vi "Test Person Updates Status on Trigger Broadcast.vi"(8 "error in (no error)":errorcluster, 11 "Person Test In":refnum<class "Person Test.lvclass">) -> (0 "error out":errorcluster, 3 "Person Test Out":refnum<class "Person Test.lvclass">)   [LabVIEW 2020, in "Person Test.lvclass"]
uses:
  Person Test.lvclass
  C:/Program Files (x86)/National Instruments/LabVIEW 2020/vi.lib/Asteme/LUnit/Test Case.lvclass
  <vilib>/Asteme/Triarc Framework/Process/Process.lvclass/Process.ctl
  <vilib>/Asteme/LUnit/Test Case.lvclass/Test Case.ctl
  <vilib>/Asteme/LUnit/LUnit Assertion Result.lvclass/LUnit Assertion Result.ctl
  <vilib>/Asteme/Triarc Framework/Process/Protected/Messaging/Enqueue Message.vi
  <vilib>/Asteme/Triarc Framework/Process/Private/SubVIs/Wait for finish.vi
  <vilib>/Asteme/Triarc Framework/Process/Private/SubVIs/Set Lifecycle State.vi
  <vilib>/Asteme/Triarc Framework/Process/Public/Lifecycle/Get Lifecycle State.vi
  <vilib>/Asteme/Triarc Framework Test Suite/Support/Execution timer.vi
  <vilib>/Asteme/LUnit/Palette/Fail.vi
  <vilib>/Asteme/LUnit/Palette/Pass.vi
  <vilib>/Asteme/LUnit/Variant to string.vi
  <vilib>/Asteme/LUnit/Set Assertion Type.vi
  <vilib>/AdvancedString/1D String Array to Delimited String.vi
  <vilib>/Utility/error.llb/Clear Errors.vi
  <vilib>/Asteme/LUnit/Add test result.vi
  <vilib>/Asteme/LUnit/LUnit Write Passed.vi
  <vilib>/Asteme/LUnit/LUnit Get Test Case.vi
  <vilib>/Asteme/LUnit/Assertion Result/LUnit Get Test Name.vi
  <vilib>/Asteme/LUnit/LUnit Write Message.vi
  <vilib>/Asteme/LUnit/LUnit Write Description.vi
  <vilib>/Asteme/LUnit/LUnit Write Assertion Type.vi
  <vilib>/Asteme/LUnit/Read Test Case Name.vi
  Person/Person.lvclass
  C:/Program Files (x86)/National Instruments/LabVIEW 2020/vi.lib/Asteme/Triarc Framework/Process/Process.lvclass
  <vilib>/Utility/error.llb/Error Cluster From Error Code.vi
  <vilib>/Asteme/Triarc Framework Test Suite/Support/Event Helpers/Dequeue Event Message.vi
  <vilib>/Utility/Data Type/Get Type Information.vi
  <vilib>/Utility/LVClass/Get LV Class Name.vi
  <vilib>/Asteme/LUnit/LUnit Assertion Result.lvclass
  <vilib>/Asteme/Triarc Framework/Process/Process.lvclass
  <vilib>/Asteme/Triarc Framework Test Suite/Support/Event Helpers/Event Helpers.lvlib
  <vilib>/Asteme/LUnit/Test Case.lvclass
  C:/Program Files (x86)/National Instruments/LabVIEW 2020/vi.lib/Asteme/Triarc Framework/View/View.lvclass
  C:/Program Files (x86)/National Instruments/LabVIEW 2020/vi.lib/Asteme/Triarc Framework/Base/Base.lvclass
  C:/Program Files (x86)/National Instruments/LabVIEW 2020/vi.lib/Asteme/Triarc Framework/Error Handler Interface/Error Handler Interface.lvclass
  C:/Program Files (x86)/National Instruments/LabVIEW 2020/vi.lib/Asteme/Triarc Framework/Logging/Logging.lvclass
  C:/Users/anton/Documents/GitHub/Triarc-Examples/Coffee Shop/Person/Person.lvclass
  C:/Program Files (x86)/National Instruments/LabVIEW 2020/vi.lib/Asteme/Triarc Framework Test Suite/View Test/View Test.lvclass
  C:/Program Files (x86)/National Instruments/LabVIEW 2020/vi.lib/Asteme/Triarc Framework Test Suite/Process Test/Process Test.lvclass
  C:/Program Files (x86)/National Instruments/LabVIEW 2020/vi.lib/Asteme/Triarc Framework Test Suite/Base Class Test/Base Test.lvclass
  C:/Users/anton/Documents/GitHub/Triarc-Examples/Coffee Shop/Person Test/Person Test.lvclass
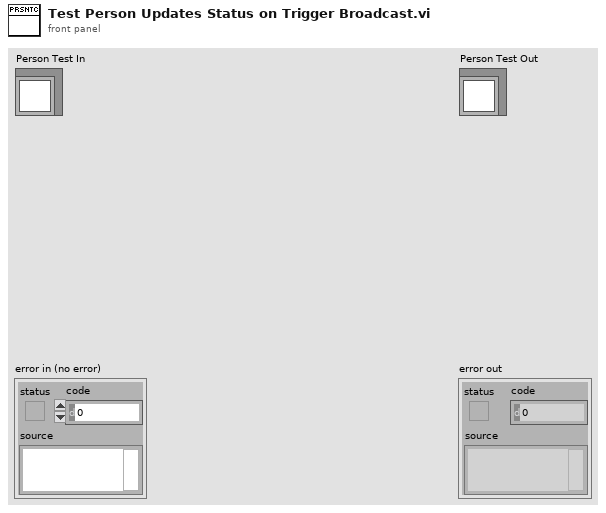
[diagram p1: front panel]
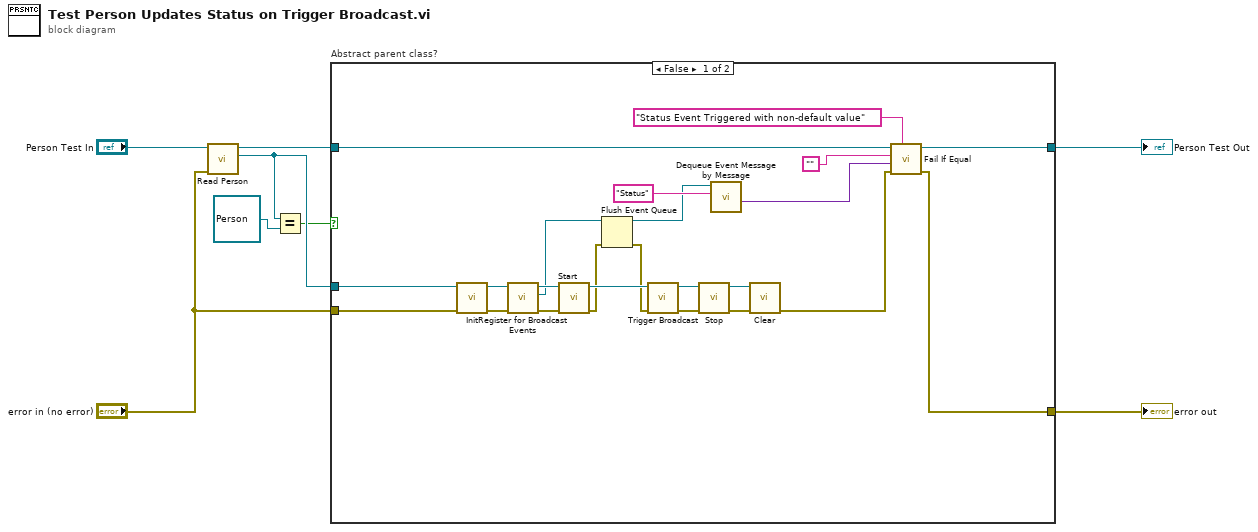
[diagram p0: block diagram]
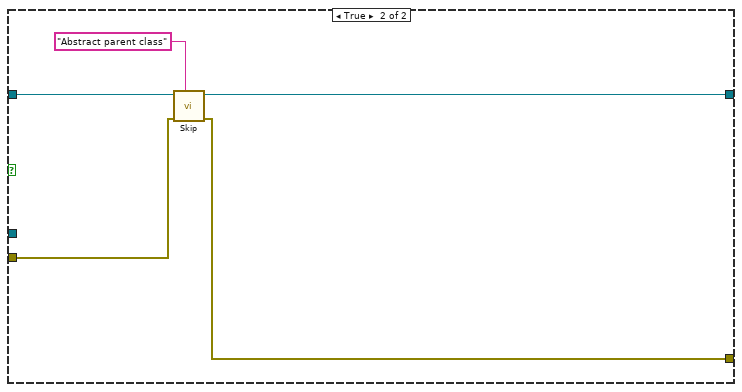
[diagram p2: hidden frame]
diagram:
  n1 = call "Read Person.vi"("error in (no error)"="error in (no error)", "Person Test in"="Person Test In") -> ("Person.lvclass"=w2:refnum<class "Person.lvclass">, "Person Test out"=w7:refnum<class "Person Test.lvclass">)  [unwired: 7 in, 1 out]
  n2 = Equal?(x=w2, y=refnum<class "Person.lvclass"> refnum ("Person.lvclass")) -> (x = y?=w1:bool)
  n3 = case "Abstract parent class?" shown="False" w1 {
    tunnel: w7 -> [w31 w36]
    tunnel: w2 -> [w20 _]
    tunnel: "error in (no error)" -> [w19 w33]
    tunnel: [w16 w35] -> w5
    tunnel: [w9 w32] -> w4
    frame False {
      n4 = call-dynamic "Init.vi"("error in (no error)"=w19, "View In"=w20) -> ("error out"=w29:errorcluster, "View Out"=w30:refnum<class "Person.lvclass">)  [unwired: 8 in]
      n5 = call <vilib>:"Register for Broadcast Events.vi"("error in (no error)"=w29, "Process In"=w30) -> ("error out"=w27:errorcluster, "Event Registration Refnum Out"=w17:refnum<event-registration>, "Process Out"=w28:refnum<class "Person.lvclass">)  [unwired: 7 in]
      n6 = call <vilib>:"Start.vi"("error in (no error)"=w27, "Process In"=w28) -> ("error out"=w25:errorcluster, "Process Out"=w26:refnum<class "Person.lvclass">)  [unwired: 8 in]
      n7 = Flush Event Queue(0:w17, 3:w25) -> (8:w11:refnum<event-registration>, 11:w18:errorcluster)  [unwired: 4 in, 1 out]
      n8 = call <vilib>:"Trigger Broadcast.vi"("error in (no error)"=w18, "Process in"=w26) -> ("error out"=w23:errorcluster, "Process out"=w24:refnum<class "Person.lvclass">)  [unwired: 8 in]
      n9 = call <vilib>:"Stop.vi"("error in (no error)"=w23, "Process In"=w24) -> ("error out"=w21:errorcluster, "Process Out"=w22:refnum<class "Person.lvclass">)  [unwired: 7 in, 1 out]
      n10 = call <vilib>:"Dequeue Event Message by Message.vi"("Message"="Status", "Event Registration Refnum"=w11) -> ("Message Data"=w13:variant)  [unwired: 5 in, 4 out]
      n11 = call-dynamic "Clear.vi"("error in (no error)"=w21, "View In"=w22) -> ("error out"=w10:errorcluster)  [unwired: 9 in]
      n12 = call <vilib>:"Fail If Equal.vi"("Description"="Status Event Triggered with non-default value", "error in (no error)"=w10, "Actual"=w13, "Expected"="", "Test Case In"=w31) -> ("error out"=w9:errorcluster, "Test Case Out"=w16:refnum<class "Person Test.lvclass">)  [unwired: 5 in]
    }
    frame True {
      n13 = call <vilib>:"Skip.vi"("Description"="Abstract parent class", "error in (no error)"=w33, "Test Case In"=w36) -> ("error out"=w32:errorcluster, "Test Case Out"=w35:refnum<class "Person Test.lvclass">)  [unwired: 7 in]
    }
  }
  "error out" <- w4
  "Person Test Out" <- w5
